vi "Set Acq Status Event.vi"(11 "statusEvent":u32) -> (2 "function return":u32, 3 "statusEvent out":u32)   [LabVIEW 2018, in "AndorSDK.lvlib"]
doc: "EXPNETTYPE unsigned int WINAPI SetAcqStatusEvent(HANDLE statusEvent);"
uses:
  AndorSDK.lvlib
  ATMCD32D.dll
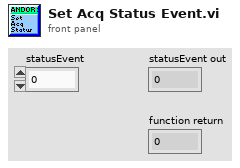
[diagram p1: front panel]
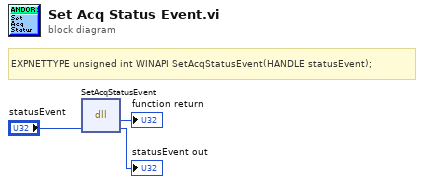
[diagram p0: block diagram]
diagram:
  # "EXPNETTYPE unsigned int WINAPI SetAcqStatusEvent(HANDLE statusEvent);"
  n1 = dll-call lib="PTH2babs E\nPersönliches02 - Arbeit03-HiwijobsLabviewCodelibANDOR\tAndor SDK\nATMCD32D.*" fn="SetAcqStatusEvent"("statusEvent"="statusEvent") -> (→"function return":u32, "statusEvent"=→"statusEvent out":u32)  [unwired: 3 in, 2 out]
